vi "Simple Reader.vi"(8 "error in (no error)":errorcluster, 11 "LabJack Driver in":refnum<class "LabJack Driver.lvclass">) -> (0 "error out":errorcluster, 2 "Signals":dbl[](array[numeric]), 3 "LabJack Driver out":refnum<class "LabJack Driver.lvclass">)   [LabVIEW 2021, in "LabJack Driver.lvclass"]
uses:
  LabJack Driver.lvclass
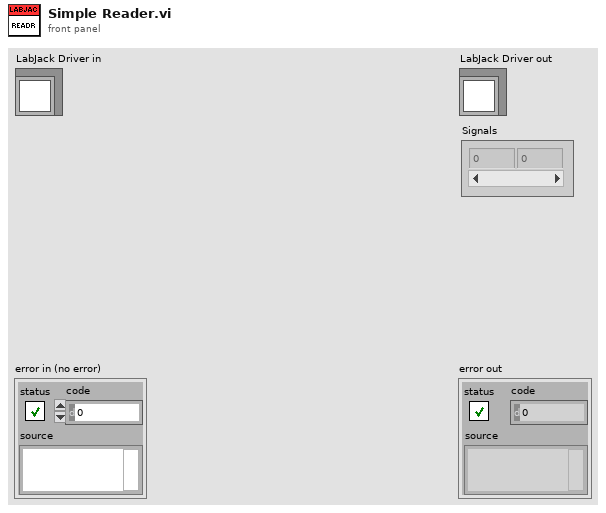
[diagram p1: front panel]
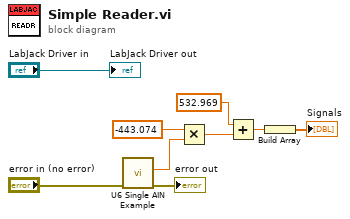
[diagram p0: block diagram]
diagram:
  n1 = call <vilib>:"U6 Single AIN Example.vi"("error in"="error in (no error)") -> ("error out"=→"error out":errorcluster, "Value Read"=w5:dbl)  [unwired: 9 in]
  n2 = Multiply(x=-443.074, y=w5) -> (x*y=w3:dbl)
  n3 = Add(x=532.969, y=w3) -> (x+y=w2:dbl)
  n4 = Build Array(w2) -> (→"Signals":dbl[])
  "LabJack Driver out" <- "LabJack Driver in"
